vi "FPGA GV.vi"() -> ()   [LabVIEW 2021]
panel:
  out "FPGA VI Reference Out":refnum<k20>
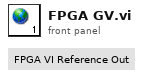
[diagram p1: front panel]
diagram:
